vi "Environmental loop.vi"(5 "Soak time (min)":dbl, 7 "Temperature (C)":string="25", 10 "Synchronized step":bool, 11 "Available PSU's":T2[](array[typedef])) -> (3 "Temperature control array":T1)   [LabVIEW 2020]
uses:
  Test Framework/Controls/PSU setting UI.ctl
  Test Framework/Controls/Temperature and voltage array.ctl
  Test Framework/Test Framework.lvclass
panel:
  out "Total number of PSU cases":i32
  out "Array 3":i32[][](array[numeric])
  out "Array 2":dbl[][](array[numeric])
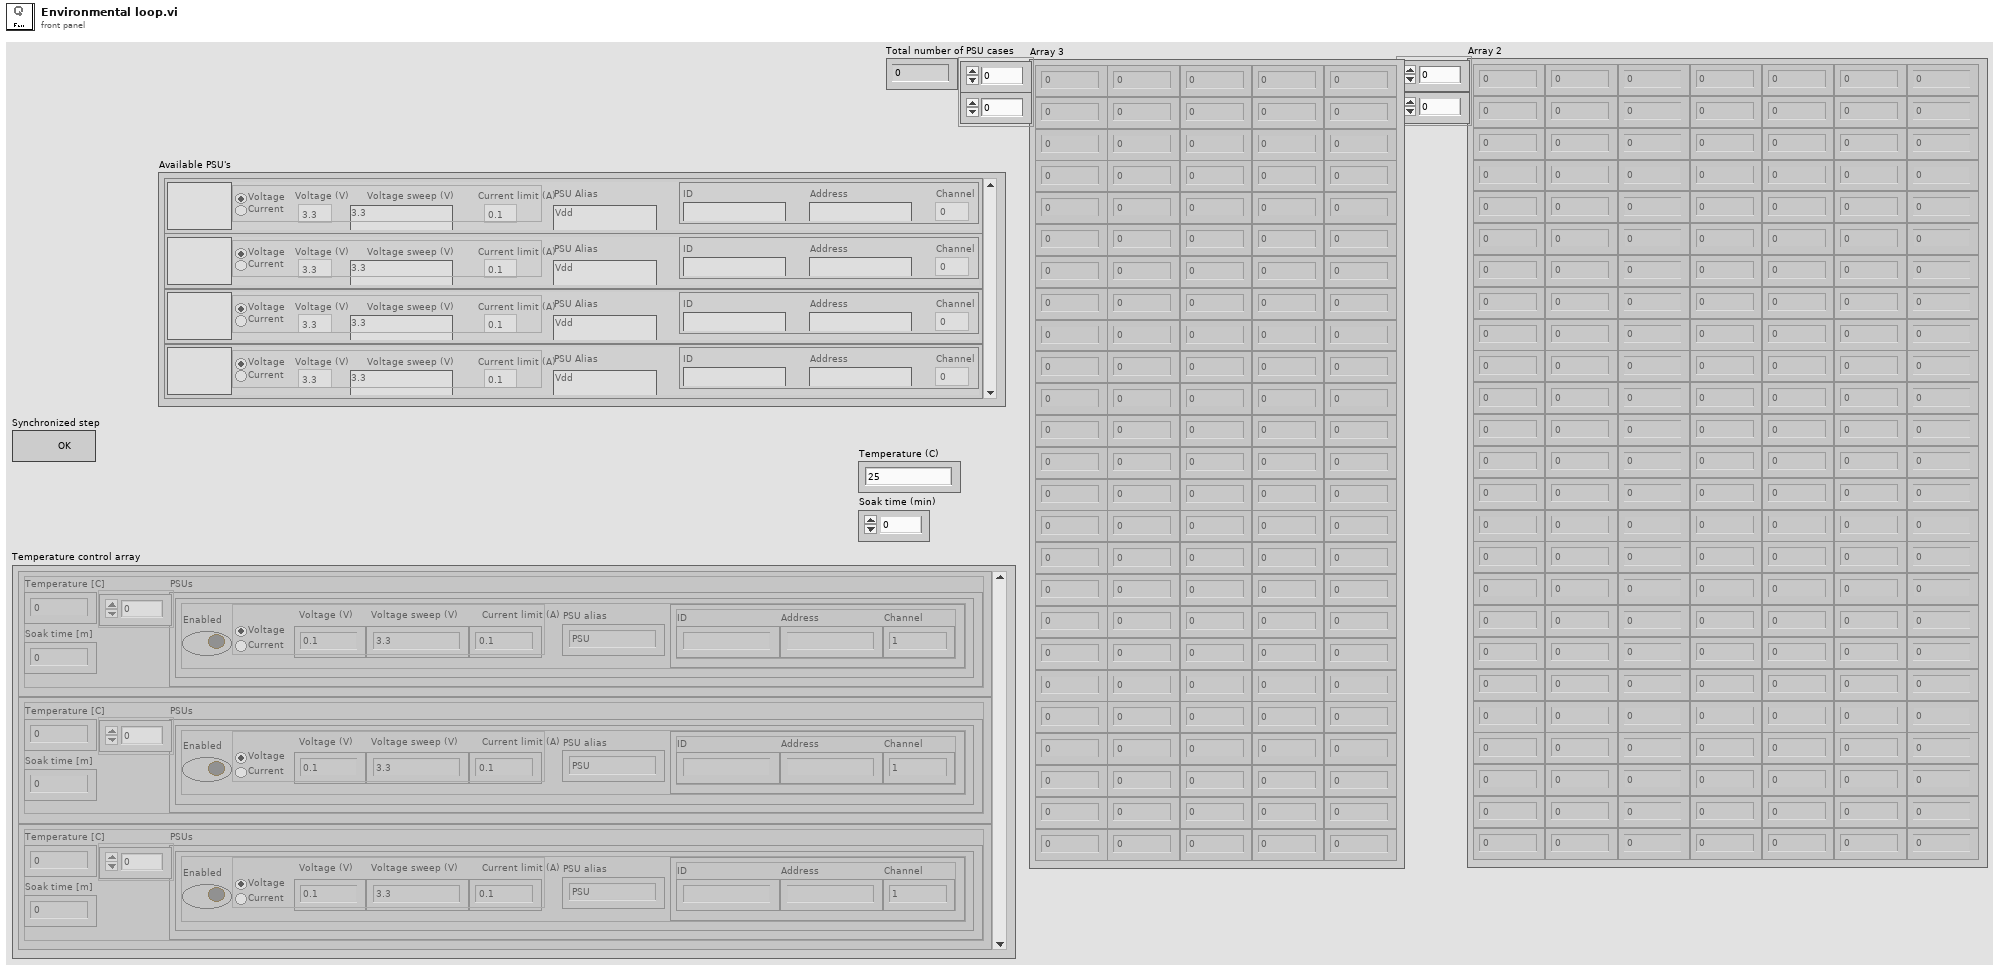
[diagram p1: front panel]
types:
  T1 = typedef "Test Framework.lvclass/Temperature and voltage array.ctl" = cluster{"Temperature [C]":dbl, "Soak time [m]":dbl, "PSUs":cluster{"Enabled":bool, "Source":enum32{"Voltage", "Current"}, "Drive (V/A)":dbl, "Sweep (V/A)":string, "Limit (A/V)":dbl, "PSU alias":string, "PSU info":cluster{"ID":string, "Address":string, "Channel":u8}}[]}[]
  T2 = typedef "Test Framework.lvclass/PSU setting UI.ctl" = cluster{"Enabled":bool, "Source":enum32{"Voltage", "Current"}, "Drive (V/A)":dbl, "Sweep (V/A)":string, "Limit (A/V)":dbl, "PSU Alias":string, "PSU info":cluster{"ID":string, "Address":string, "Channel":u8}}
  T3 = cluster{"Temperature [C]":dbl, "Soak time [m]":dbl, "PSUs":cluster{"Enabled":bool, "Source":enum32{"Voltage", "Current"}, "Drive (V/A)":dbl, "Sweep (V/A)":string, "Limit (A/V)":dbl, "PSU alias":string, "PSU info":cluster{"ID":string, "Address":string, "Channel":u8}}[]}
  T4 = cluster{"Enabled":bool, "Source":enum32{"Voltage", "Current"}, "Drive (V/A)":dbl, "Sweep (V/A)":string, "Limit (A/V)":dbl, "PSU alias":string, "PSU info":cluster{"ID":string, "Address":string, "Channel":u8}}
  T5 = cluster{"Numeric":dbl, "Soak time (min)":dbl, "Available PSU's":T2[]}
  T6 = cluster{"Numeric":dbl, "Soak time (min)":dbl, "Available PSU's":T2[]}[]
  T7 = cluster{"Temperature [C]":dbl, "Soak time [m]":dbl, "PSUs":T2[]}[]
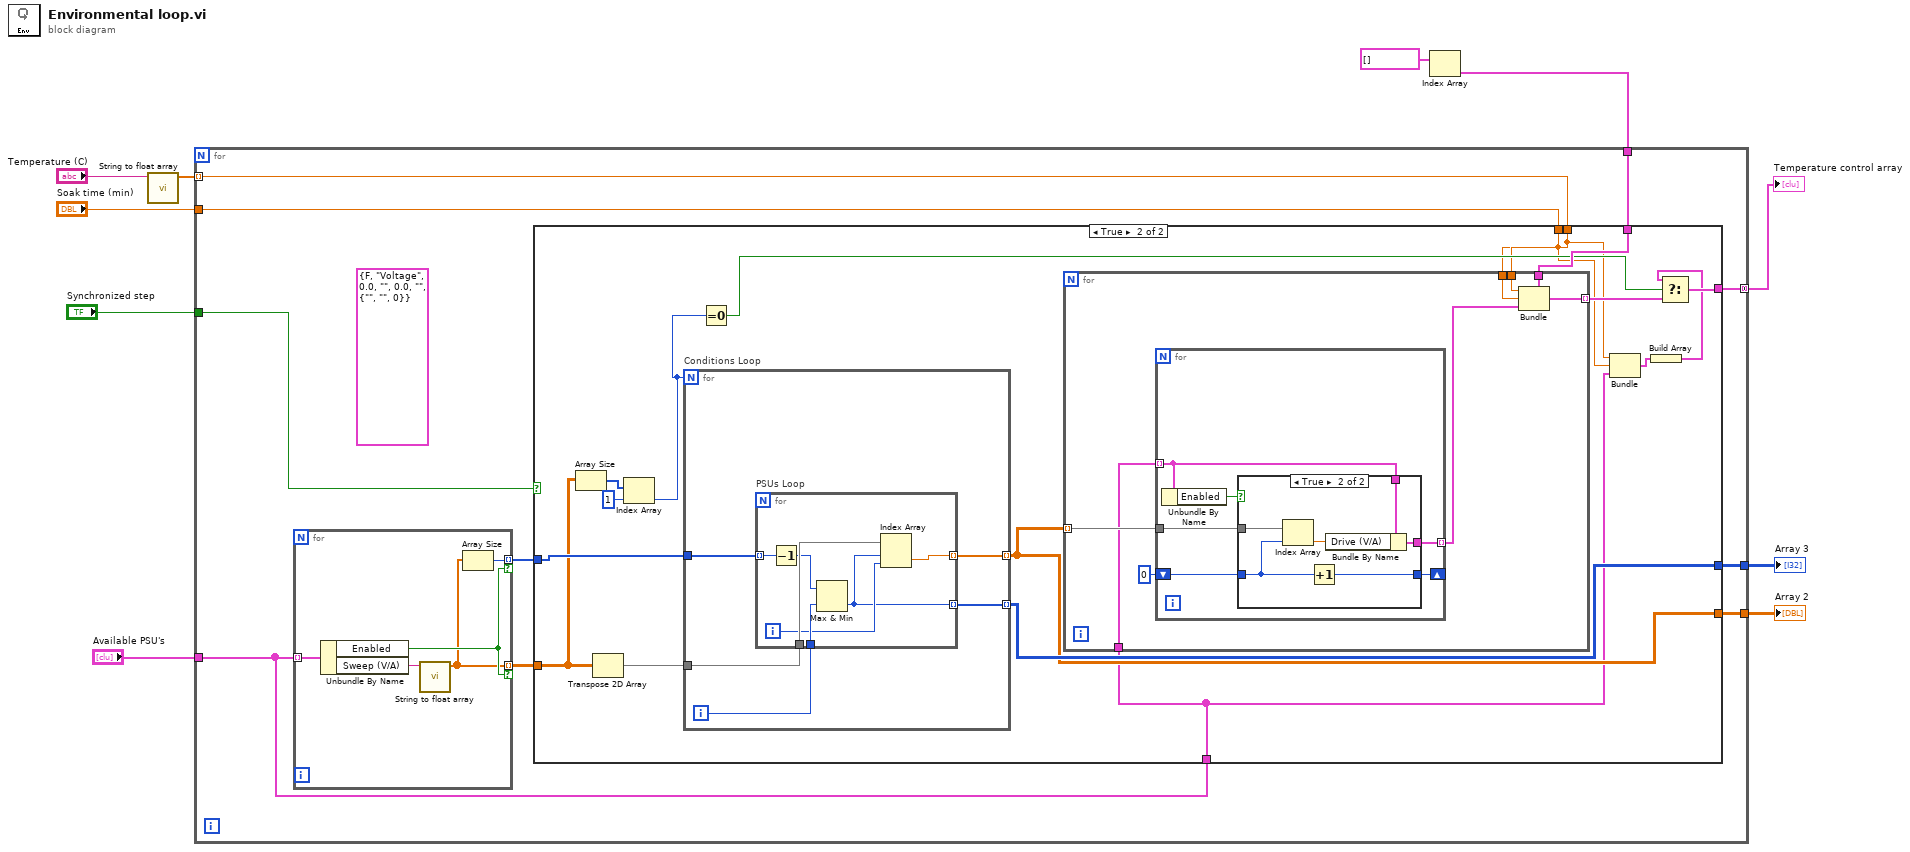
[diagram p0: block diagram]
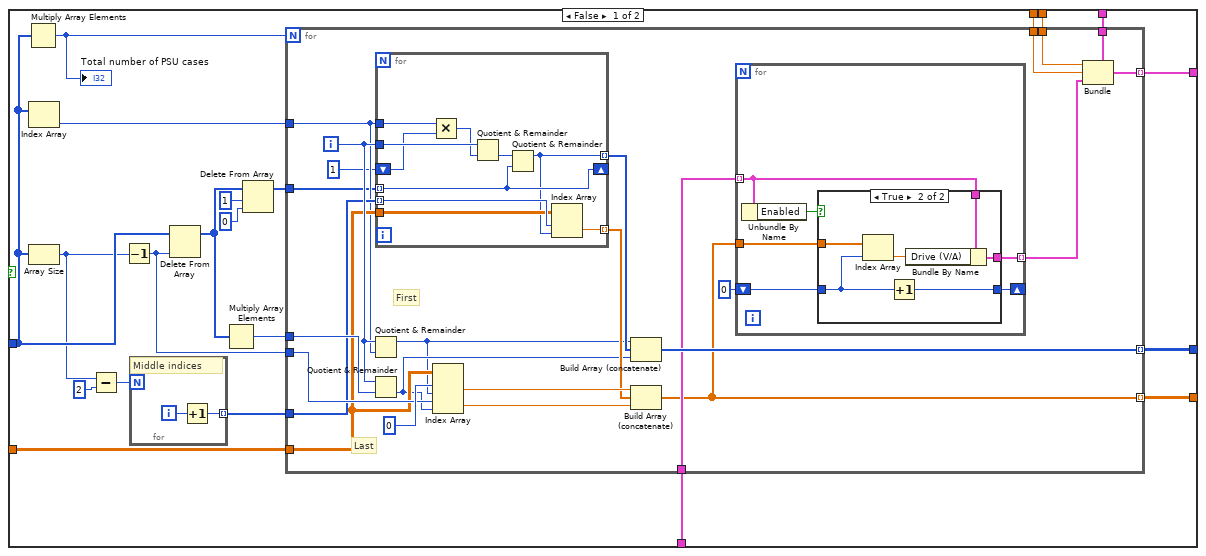
[diagram p2: hidden frame]
diagram:
  n1 = call "String to float array.vi"("String"="Temperature (C)") -> ("Array - Numeric"=w7:dbl[])  [unwired: 9 in, 1 out]
  n2 = Index Array(array=T1 [] ("Temperature control array")) -> (element=w4:T3)  [unwired: 1 in]
  n3 = for {
    tunnel: "Available PSU's" -> [w12]
    tunnel: w7 -> [w15] mode=indexing
    tunnel: [w18] -> w6
    tunnel: [w17] -> w5
    tunnel: w4 -> [w16]
    tunnel: "Soak time (min)" -> [w14]
    tunnel: [w13] -> w2 mode=concatenating
    tunnel: "Synchronized step" -> [w11]
    (unwired) T4 {"Enabled"=FALSE, "Source"=enum."Voltage", "Drive (V/A)"=0.0, "Sweep (V/A)"="", "Limit (A/V)"=0.0, "PSU alias"="", "PSU info"={"ID"="", "Address"="", "Channel"=0}} ("PSU")
    n4 = for {
      tunnel: [w144] -> w20 mode=indexing if=w145
      tunnel: [w143] -> w19 mode=indexing if=w145
      tunnel: w12 -> [w146] mode=indexing
      n5 = Unbundle By Name(w146) -> ("Enabled"=w145:bool, "Sweep (V/A)"=w147:string)
      n6 = call "String to float array.vi"("String"=w147) -> ("Array - Numeric"=w144:dbl[])  [unwired: 9 in, 1 out]
      n7 = Array Size(array=w144) -> (size(s)=w143:i32)
    }
    n8 = case shown="True" w11 {
      tunnel: w20 -> [w41 w104]
      tunnel: w19 -> [w38 w107]
      tunnel: [w27 w106] -> w18
      tunnel: [w26 w105] -> w17
      tunnel: w16 -> [w25 w100]
      tunnel: w15 -> [w24 w94]
      tunnel: w14 -> [w23 w93]
      tunnel: [w22 w97] -> w13
      tunnel: w12 -> [w21 w92]
      frame False {
        n9 = Multiply Array Elements(1:w38) -> (0:w36:i32)
        "Total number of PSU cases" <- w36
        n10 = Index Array(array=w38) -> (element=w37:i32)  [unwired: 1 in]
        n11 = Array Size(array=w38) -> (size(s)=w35:i32)
        n12 = Subtract(x=w35, y=2) -> (x-y=w33:i32)
        n13 = Decrement(x=w35) -> (x-1=w40:i32)
        n14 = for {
          N: w33 -> [_]
          tunnel: [w42] -> w32 mode=indexing
          i -> [w43]
          # "Middle indices"
          n15 = Increment(x=w43) -> (x+1=w42:i32)
        }
        n16 = Delete From Array(array=w38, index=w40) -> (array with subset deleted=w31:i32[])  [unwired: 1 in, 1 out]
        n17 = Multiply Array Elements(1:w31) -> (0:w39:i32)
        n18 = Delete From Array(array=w31, length=1, index=0) -> (array with subset deleted=w28:i32[])  [unwired: 1 out]
        n19 = for {
          N: w36 -> [_]
          tunnel: w41 -> [w60]
          tunnel: w37 -> [w58]
          tunnel: [w46] -> w26 mode=indexing
          tunnel: [w52] -> w27 mode=indexing
          tunnel: w40 -> [w63]
          tunnel: w39 -> [w65]
          tunnel: w32 -> [w61]
          tunnel: w28 -> [w57]
          tunnel: w25 -> [w51]
          tunnel: w24 -> [w50]
          tunnel: w23 -> [w49]
          tunnel: [w48] -> w22 mode=indexing
          tunnel: w21 -> [w47]
          i -> [w62]
          # "Last"
          # "First"
          n20 = Quotient & Remainder(x=w62, y=w58) -> (x-y*floor(x/y)=w53:i32)  [unwired: 1 out]
          n21 = Quotient & Remainder(x=w62, y=w65) -> (floor(x/y)=w54:i32)  [unwired: 1 out]
          n22 = for {
            tunnel: w62 -> [w91]
            tunnel: w57 -> [w86] mode=indexing
            tunnel: w61 -> [w90] mode=indexing
            tunnel: w60 -> [w89]
            tunnel: [w88] -> w59 mode=indexing
            shift-right: [w86] -> _
            shift-left: 1 -> [w85]
            tunnel: [w82] -> w55 mode=indexing
            tunnel: w58 -> [w84]
            n23 = Multiply(x=w84, y=w85) -> (x*y=w83:i32)
            n24 = Quotient & Remainder(x=w91, y=w83) -> (floor(x/y)=w87:i32)  [unwired: 1 out]
            n25 = Quotient & Remainder(x=w87, y=w86) -> (x-y*floor(x/y)=w82:i32)  [unwired: 1 out]
            n26 = Index Array(array=w89, index (row)=w90, index (col)=w82) -> (element=w88:dbl)
          }
          n27 = Index Array(array=w60, index (row) #1=0 ("disabled index (col)"), index (col) #1=w53, index (row) #2=w63, index (col) #2=w54) -> (element #1=w67:dbl, element #2=w66:dbl)
          n28 = Build Array (concatenate)(w53, w55, w54) -> (w52:i32[])
          n29 = Build Array (concatenate)(w67, w59, w66) -> (w46:dbl[])
          n30 = for {
            tunnel: w47 -> [w72] mode=indexing
            tunnel: w46 -> [w73]
            tunnel: [w70] -> w45 mode=indexing
            shift-right: [w68] -> _
            shift-left: 0 -> [w69]
            n31 = Unbundle By Name(w72) -> ("Enabled"=w71:bool)
            n32 = case shown="True" w71 {
              tunnel: w73 -> [_ w78]
              tunnel: w72 -> [w75 w81]
              tunnel: [w75 w80] -> w70
              tunnel: w69 -> [w74 w77]
              tunnel: [w74 w76] -> w68
              frame False {
              }
              frame True {
                n33 = Index Array(array=w78, index=w77) -> (element=w79:dbl)
                n34 = Increment(x=w77) -> (x+1=w76:i32)
                n35 = Bundle By Name(cluster=w81, "Drive (V/A)"=w79) -> (w80:T2)
              }
            }
          }
          n36 = Bundle(cluster=w51, "Temperature [C]"=w50, "Soak time [m]"=w49, "PSUs"=w45) -> (w48:T3)
        }
      }
      frame True {
        n37 = Array Size(array=w104) -> (size(s)=w103:i32[])
        n38 = Transpose 2D Array(2D array=w104) -> (transposed array=w108:dbl[][])
        n39 = Index Array(array=w103, index=1) -> (element=w101:i32)
        n40 = for "Conditions Loop" {
          N: w101 -> [_]
          tunnel: w108 -> [w135]
          tunnel: w107 -> [w133]
          tunnel: [w132] -> w105 mode=indexing
          tunnel: [w131] -> w106 mode=indexing
          i -> [w134]
          n41 = for "PSUs Loop" {
            tunnel: w135 -> [w142]
            tunnel: w134 -> [w141]
            tunnel: w133 -> [w138] mode=indexing
            tunnel: [w140] -> w132 mode=indexing
            tunnel: [w136] -> w131 mode=indexing
            i -> [w139]
            n42 = Decrement(x=w138) -> (x-1=w137:i32)
            n43 = Max & Min(x=w137, y=w141) -> (min(x,y)=w136:i32)  [unwired: 1 out]
            n44 = Index Array(array=w142, index (row)=w136, index (col)=w139) -> (element=w140:dbl)
          }
        }
        n45 = Equal To 0?(x=w101) -> (x = 0?=w99:bool)
        n46 = for {
          tunnel: w100 -> [w116]
          tunnel: w94 -> [w115]
          tunnel: w93 -> [w114]
          tunnel: [w113] -> w98 mode=indexing
          tunnel: w105 -> [w111] mode=indexing
          tunnel: w92 -> [w110]
          n47 = for {
            tunnel: w110 -> [w121] mode=indexing
            tunnel: w111 -> [w122]
            tunnel: [w119] -> w109 mode=indexing
            shift-right: [w117] -> _
            shift-left: 0 -> [w118]
            n48 = Unbundle By Name(w121) -> ("Enabled"=w120:bool)
            n49 = case shown="True" w120 {
              tunnel: w122 -> [_ w127]
              tunnel: w121 -> [w124 w130]
              tunnel: [w124 w129] -> w119
              tunnel: w118 -> [w123 w126]
              tunnel: [w123 w125] -> w117
              frame False {
              }
              frame True {
                n50 = Index Array(array=w127, index=w126) -> (element=w128:dbl)
                n51 = Increment(x=w126) -> (x+1=w125:i32)
                n52 = Bundle By Name(cluster=w130, "Drive (V/A)"=w128) -> (w129:T2)
              }
            }
          }
          n53 = Bundle(cluster=w116, "Temperature [C]"=w115, "Soak time [m]"=w114, "PSUs"=w109) -> (w113:T3)
        }
        n54 = Bundle("Numeric"=w94, "Soak time (min)"=w93, "Available PSU's"=w92) -> (w96:T5)  [unwired: 1 in]
        n55 = Build Array(w96) -> (w95:T6)
        n56 = Select(t=w95, s=w99, f=w98) -> (s? t:f=w97:T7)
      }
    }
  }
  "Temperature control array" <- w2
  "Array 2" <- w5
  "Array 3" <- w6
